vi "Get_Temperature.vi"(0 "error in":errorcluster) -> (1 "error out":errorcluster, 2 "Temperature":dbl)   [LabVIEW 2010]
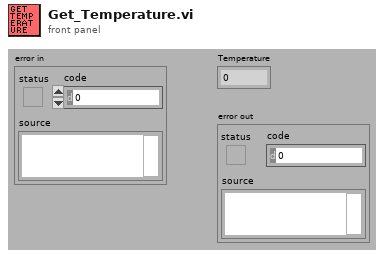
[diagram p1: front panel]
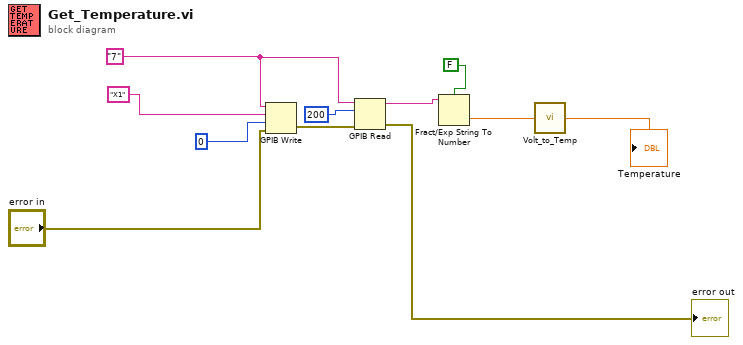
[diagram p0: block diagram]
diagram:
  w4 = "7"
  n1 = GPIB Write(0:w4, 1:"X1", 2:0, 3:"error in") -> (6:w7:errorcluster)  [unwired: 1 in, 1 out]
  n2 = GPIB Read(0:w4, 1:200, 3:w7) -> (5:w3:string, 7:→"error out":errorcluster)  [unwired: 2 in, 1 out]
  n3 = Fract/Exp String To Number(use system decimal point (T)=FALSE, string=w3) -> (number=w1:dbl)  [unwired: 2 in, 1 out]
  n4 = call "Volt_to_Temp.vi"("Voltage"=w1) -> ("Temperature"=→"Temperature":dbl)
